vi "MQTT_PubRel_Read.vi"(8 "error in (no error)":errorcluster, 11 "connection ID":refnum<k5>) -> (0 "error out":errorcluster, 2 "Message ID":u16=10 format="%x", 3 "connection ID out":refnum<k5>)   [LabVIEW 2025, in "DAQIO MQTT.lvlib"]
doc: "© 2015 - daq.io, LLC - Peter Adelhardt"
uses:
  DAQIO MQTT.lvlib
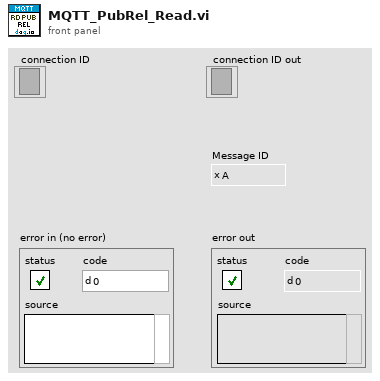
[diagram p1: front panel]
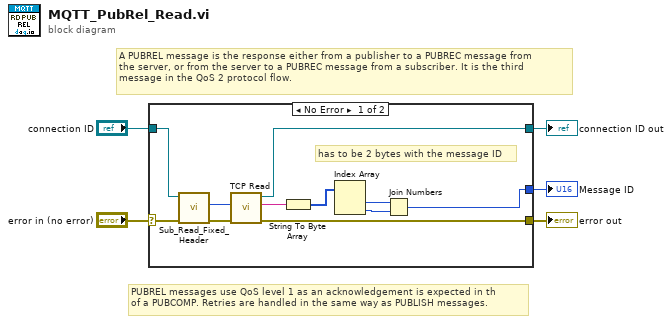
[diagram p0: block diagram]
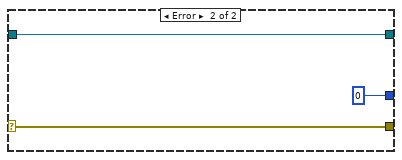
[diagram p2: hidden frame]
diagram:
  # "PUBREL messages use QoS level 1 as an acknowledgement is expected in th\nof a PUBCOMP. Retries are handled in the same way as PUBLISH messages."
  # "A PUBREL message is the response either from a publisher to a PUBREC message from\nthe server, or from the server to a PUBREC message from a subscriber. It is the third\nmessage in the QoS 2 protocol flow."
  n1 = case shown="No Error" "error in (no error)" {
    selector: "error in (no error)" -> [w15 w19]
    tunnel: [w9 w19] -> w4
    tunnel: [w8 w18] -> w3
    tunnel: [w7 u16 0] -> w2
    tunnel: "connection ID" -> [w6 w18]
    frame No Error {
      # "has to be 2 bytes with the message ID"
      n2 = call "Sub_Read_Fixed_Header.vi"("error in (no error)"=w15, "connection ID"=w6) -> ("error out"=w10:errorcluster, "Remaining Length"=w16:u32)  [unwired: 3 in, 5 out]
      n3 = call "TCP Read.vi"("error in (no error)"=w10, "bytes to read"=w16) -> ("error out"=w9:errorcluster, "data out"=w11:string, "connection ID out"=w8:refnum<k5>)  [unwired: 7 in]
      n4 = String To Byte Array(string=w11) -> (unsigned byte array=w12:u8[])
      n5 = Index Array(array=w12) -> (element #1=w14:u8, element #2=w13:u8)  [unwired: 2 in]
      n6 = Join Numbers(hi=w14, lo=w13) -> ((hi.lo)=w7:u16)
    }
    frame Error {
    }
  }
  "error out" <- w4
  "Message ID" <- w2
  "connection ID out" <- w3
